vi "Tell Parent Init.vi"(7 "Actor in":refnum<class "Actor.lvclass">, 9 "Msg Attributes":T1 {"Teller"."Absolute Time" format="%<%x %.3X>T"}) -> (0 "Error out":errorcluster, 1 "Told":bool, 5 "Actor out":refnum<class "Actor.lvclass">)   [LabVIEW 2020, in "jettl.lvlib"]
uses:
  jettl.lvlib
  Actor/Actor.lvclass
  Msg Input/Msg Input.lvclass
  Msg Output/Msg Output.lvclass
  Msg/Msg.lvclass
  Relation.ctl
  Teller.ctl
  Msg Attributes.ctl
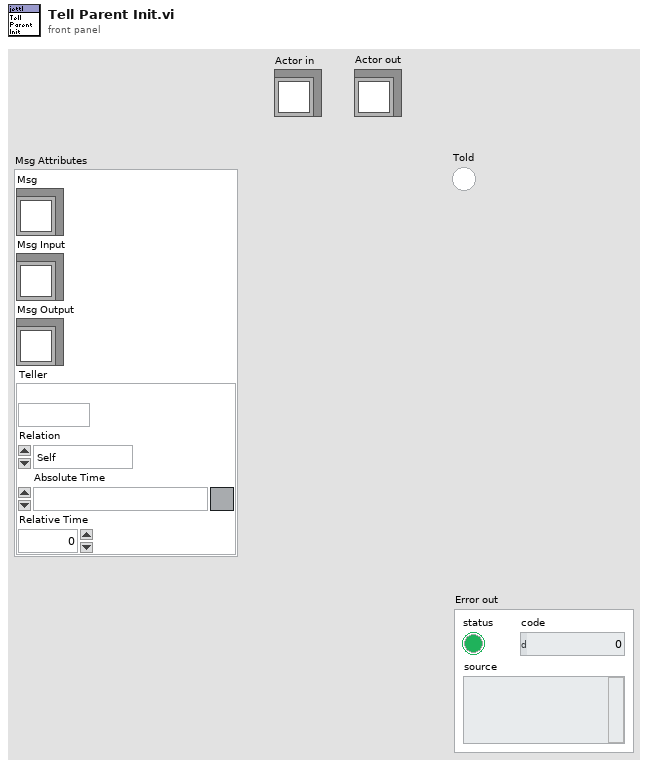
[diagram p1: front panel]
types:
  T1 = typedef "jettl.lvlib/Msg Attributes.ctl" = cluster{"Msg":refnum<class "Msg.lvclass">, "Msg Input":refnum<class "Msg Input.lvclass">, "Msg Output":refnum<class "Msg Output.lvclass">, "Teller":T2}
  T2 = typedef "jettl.lvlib/Teller.ctl" = cluster{"Alias":string, "Relation":T3, "Absolute Time":timestamp, "Relative Time":dbl}
  T3 = typedef "jettl.lvlib/Relation.ctl" = enum16{"Self", "Parent", "Child"}
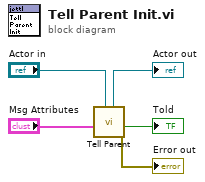
[diagram p0: block diagram]
diagram:
  n1 = call "Tell Parent.vi"("Actor in"="Actor in", "Msg Attributes"="Msg Attributes") -> ("Error out"=→"Error out":errorcluster, "Told"=→"Told":bool, "Actor out"=→"Actor out":refnum<class "Actor.lvclass">)  [unwired: 7 in]
